vi "MQTT_Read_Subscribed_Topics.vi"(8 "error in (no error)":errorcluster) -> (0 "error out":errorcluster)   [LabVIEW 2018, in "MQTT_Functions.lvlib"]
uses:
  MQTT_Functions.lvlib
  Controls/QoS.ctl
  Controls/Connect_Flags.ctl
  Controls/Retain_Flag.ctl
  Controls/DUP_Flag.ctl
  Controls/User_Info.ctl
  Controls/Connection_Return_Codes.ctl
panel:
  out "Connection Status":T1=enum."Connection refused: not authorized"
  in  "Exit":bool
  in  "MQTT Broker":cluster{"address (IP)":string, "port":u16}={"address (IP)"="green.daqloud.com", "port"=1883}
  out "Message IDs":u16[](array[numeric]) format="%x"
  out "Topics":string[](array[string])
  out "Messages":string[](array[string])
  in  "Client ID":string="NodeE-12345"
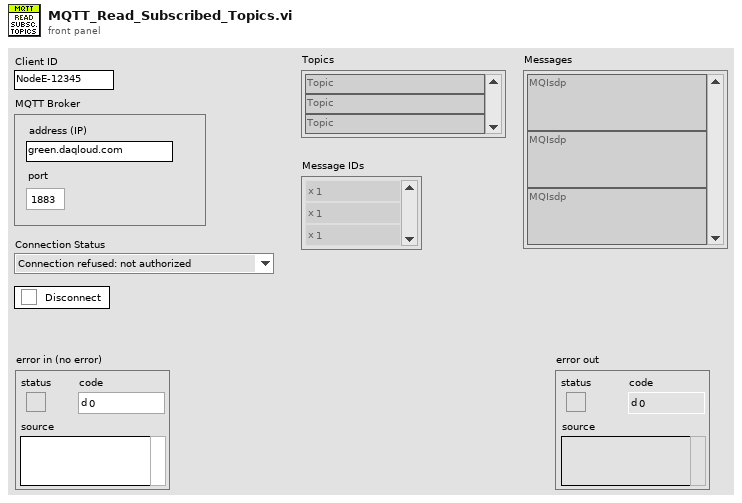
[diagram p1: front panel]
types:
  T1 = typedef "MQTT_Functions.lvlib/Connection_Return_Codes.ctl" = enum16{"Connection accepted", "Connection refused: unacceptable protocol version", "Connection refused: identifier rejected", "Connection refused: Server unavailable", "Connection refused: bad user name or password", "Connection refused: not authorized"}
  T2 = typedef "MQTT_Functions.lvlib/User_Info.ctl" = cluster{"User Name":string, "Password":string}
  T3 = typedef "MQTT_Functions.lvlib/QoS.ctl" = enum8{"At most once", "At least once", "Exactly once", "Reserved"}
  T4 = typedef "MQTT_Functions.lvlib/DUP_Flag.ctl" = bool
  T5 = typedef "MQTT_Functions.lvlib/Retain_Flag.ctl" = bool
  T6 = cluster{"QoS":T3, "DUP":T4, "Retain":T5, "Keep Alive (sec)":u16}
  T7 = typedef "MQTT_Functions.lvlib/Connect_Flags.ctl" = cluster{"user name":bool, "password":bool, "will retain":bool, "will flag":bool, "clean session":bool, "reserved":bool, "will QoS":T3}
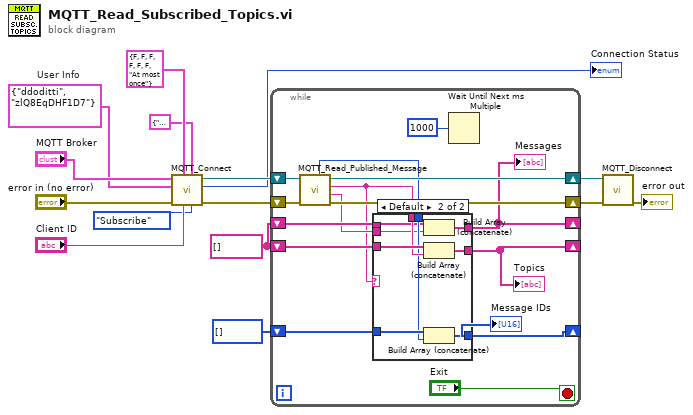
[diagram p0: block diagram]
diagram:
  w2 = T2 {"User Name"="ddoditti", "Password"="zlQ8EqDHF1D7"}  # User Info
  w8 = string[] []
  n1 = call "MQTT_Connect.vi"(4:enum16{"Publish", "Subscribe"}."Subscribe" ("Publish/Subscribe"), "Connect Meta"=T6 {"QoS"=enum."At most once", "DUP"=FALSE, "Retain"=FALSE, "Keep Alive (sec)"=60}, "Client ID"="Client ID", "Connect Flags"=T7 {"user name"=FALSE, "password"=FALSE, "will retain"=FALSE, "will flag"=FALSE, "clean session"=FALSE, "reserved"=FALSE, "will QoS"=enum."At most once"}, "error in (no error)"="error in (no error)", "User Info"=w2, "MQTT Broker"="MQTT Broker") -> ("error out"=w3:errorcluster, "Connection Status"=→"Connection Status":T1, "connection ID out"=w5:refnum<k5>)  [unwired: 2 in]
  n2 = while {
    shift-right: [w25] -> w10
    shift-left: w3 -> [w27]
    shift-right: [w17] -> _
    shift-left: u16[] [] -> [w23]
    shift-right: [w18] -> _
    shift-left: w8 -> [w21]
    shift-right: [w19] -> _
    shift-left: w8 -> [w24]
    shift-right: [w26] -> w11
    shift-left: w5 -> [w28]
    stop <- "Exit" stop-if-true
    n3 = call "MQTT_Read_Published_Message.vi"("error in (no error)"=w27, "connection ID"=w28) -> ("error out"=w25:errorcluster, "Message"=w20:string, "Topic Name"=w16:string, "connection ID out"=w26:refnum<k5>, "Message ID"=w22:u16)  [unwired: 4 in, 1 out]
    n4 = case shown="Default" w16 {
      tunnel: w24 -> [w32 w42]
      tunnel: w16 -> [_ w41]
      tunnel: w23 -> [w31 w40]
      tunnel: w22 -> [_ w39]
      tunnel: w21 -> [w33 w38]
      tunnel: w20 -> [_ w37]
      tunnel: [w32 w36] -> w19
      tunnel: [w33 w35] -> w18
      tunnel: [w31 w34] -> w17
      frame "Topic" {
      }
      frame Default {
        n5 = Build Array (concatenate)(w38, w37) -> (w35:string[])
        n6 = Build Array (concatenate)(w42, w41) -> (w36:string[])
        n7 = Build Array (concatenate)(w40, w39) -> (w34:u16[])
      }
    }
    "Topics" <- w19
    "Messages" <- w18
    "Message IDs" <- w17
    n8 = Wait Until Next ms Multiple(millisecond multiple=u32 1000) -> ()  [unwired: 1 out]
  }
  n9 = call "MQTT_Disconnect.vi"("error in (no error)"=w10, "connection ID"=w11) -> ("error out"=→"error out":errorcluster)  [unwired: 9 in]
